vi "array-to-time.vi"(2 "index":i32, 3 "Array":string[](array[string])) -> (0 "element":string, 1 "output array":string[](array[string]))   [LabVIEW 2023]
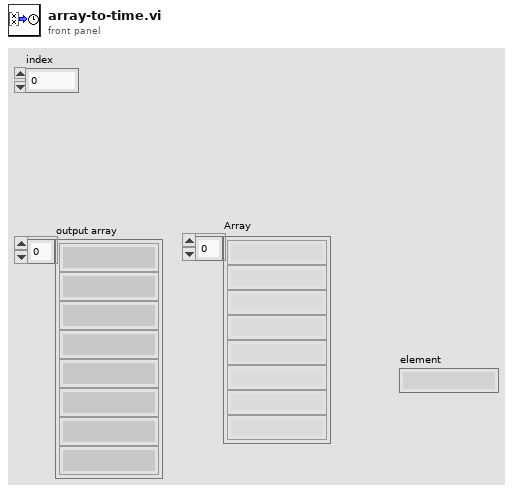
[diagram p1: front panel]
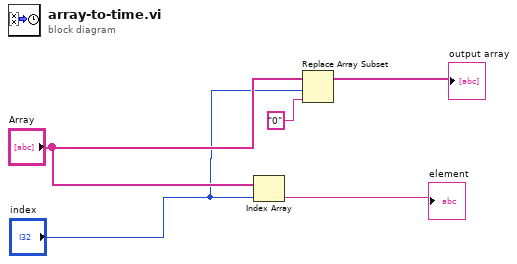
[diagram p0: block diagram]
diagram:
  n1 = Index Array(array="Array", index="index") -> (element=→"element":string)
  n2 = Replace Array Subset(array="Array", new element="0" ("new element/subarray"), index="index") -> (→"output array":string[])
